vi "_Read.vi"(8 "error in (no error)":errorcluster, 11 "Collection in":refnum<class "Collection.lvclass">) -> (0 "error out":errorcluster, 2 "X array":T1, 3 "Collection out":refnum<class "Collection.lvclass">)   [LabVIEW 2023, in "Collection.lvclass"]
doc: "(Protected, Dynamic, Pure Virtual/Abstract) Perform a measurement and return one or more channels of data. Outsiders should not call this method, but instead the public \"Read Data.vi\"."
uses:
  Collection.lvclass
  Readable/X array.ctl
  Readable/X.ctl
  Collection.lvclass/Collection.ctl
  Readable/Readable.lvclass
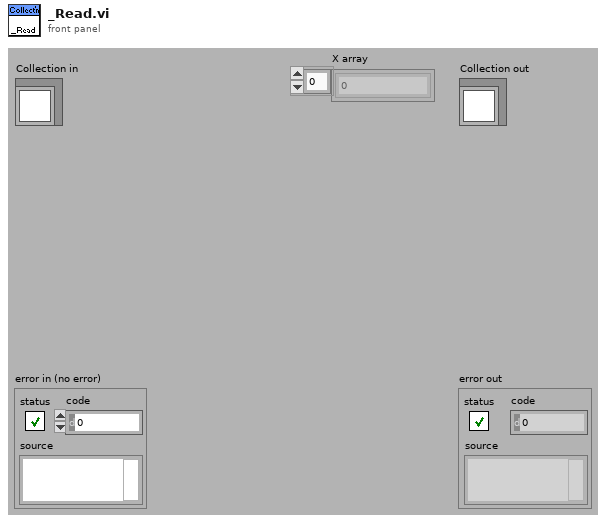
[diagram p1: front panel]
types:
  T1 = typedef "Readable.lvclass/X array.ctl" = T2[]
  T2 = typedef "Readable.lvclass/X.ctl" = dbl
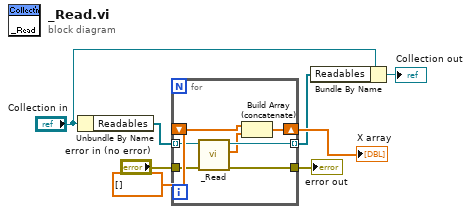
[diagram p0: block diagram]
diagram:
  n1 = Unbundle By Name("Collection in") -> ("Readables"=w7:refnum<class "Readable.lvclass">[])
  n2 = for {
    shift-right: [w14] -> w8
    shift-left: T1 [] ("X array") -> [w15]
    tunnel: w7 -> [w13] mode=indexing
    tunnel: [w12] -> w5 mode=indexing
    tunnel: "error in (no error)" -> [w11]
    tunnel: [w10] -> w2
    n3 = call-dynamic "_Read.vi"("error in (no error)"=w11, "Readable in"=w13) -> ("error out"=w10:errorcluster, "X array"=w9:T1, "Readable out"=w12:refnum<class "Readable.lvclass">)  [unwired: 7 in]
    n4 = Build Array (concatenate)(w15, w9) -> (w14:T1)
  }
  "error out" <- w2
  "X array" <- w8
  n5 = Bundle By Name(cluster="Collection in", "Readables"=w5) -> (→"Collection out":refnum<class "Collection.lvclass">)
